vi "Report Generator.vi"(8 "error in (no error)":errorcluster, 11 "Report File Path":path) -> (0 "error out":errorcluster, 3 "report out":T1)   [LabVIEW 2020, in "WebServiceImporter.lvlib" / "Error Handling.lvlib"]
uses:
  <vilib>/Platform/WebService/Error Handling/Error Handling.lvlib
  <resource>/importtools/NISH Report/Generate Report Object Reference.ctl
  <resource>/importtools/NISH Report/NISH Report.lvlib
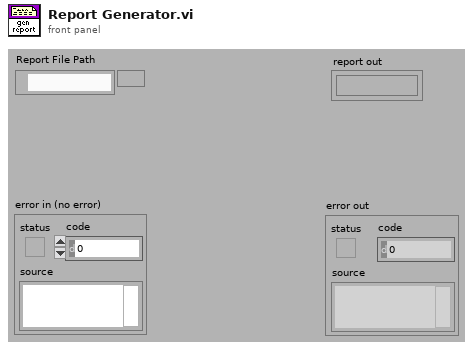
[diagram p1: front panel]
types:
  T1 = typedef "NISH Report.lvlib/Generate Report Object Reference.ctl" = refnum<k1>
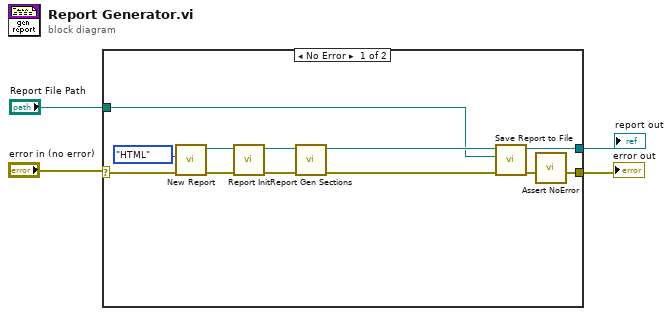
[diagram p0: block diagram]
diagram:
  n1 = case shown="No Error" "error in (no error)" {
    selector: "error in (no error)" -> [w16 w17]
    tunnel: [w5 w17] -> w3
    tunnel: [w14 _] -> w2
    tunnel: "Report File Path" -> [w7 _]
    frame No Error {
      n2 = call <resource>:"New Report.vi"("error in (no error)"=w16, "report type"=enum16{"Standard Report", "HTML"}."HTML") -> ("error out"=w13:errorcluster, "report out"=w12:T1)  [unwired: 4 in]
      n3 = call <vilib>:"Report Init.vi"("error in (no error)"=w13, "report"=w12) -> ("error out"=w11:errorcluster, "report out"=w10:T1)  [unwired: 8 in]
      n4 = call <vilib>:"Report Gen Sections.vi"("error in (no error)"=w11, "report"=w10) -> ("error out"=w9:errorcluster, "report out"=w8:T1)  [unwired: 8 in]
      n5 = call <resource>:"Save Report to File.vi"("error in (no error)"=w9, "report file path"=w7, "report in"=w8) -> ("error out"=w6:errorcluster, "report out"=w14:T1)  [unwired: 3 in]
      n6 = call <vilib>:"Assert NoError.vi"("error in (no error)"=w6) -> ("error out"=w5:errorcluster)  [unwired: 10 in]
    }
    frame Error {
    }
  }
  "error out" <- w3
  "report out" <- w2
